vi "Revive Jaguars.vi"() -> ()   [LabVIEW 2011]
uses:
  <vilib>/Rock Robotics/WPI/CAN/Jaguar/SubVIs/WPI_CANJaguar_ControlMode.ctl
  <vilib>/Rock Robotics/WPI/CAN/Jaguar/SubVIs/WPI_CANJaguar_StatusSelect.ctl
  <vilib>/Rock Robotics/WPI/CAN/Jaguar/SubVIs/WPI_CANJaguar_SpeedReference.ctl
  Globals/Robot Jaguars.vi
  <vilib>/Rock Robotics/WPI/MotorControl/WPI_MotorControlOpenCANJaguar.vi
panel:
  out "FLD Mode":T1
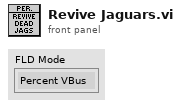
[diagram p1: front panel]
types:
  T1 = typedef "WPI_CANJaguar_ControlMode.ctl" = enum8{"Percent VBus", "Current", "Speed", "Position", "Voltage"}
  T2 = typedef "WPI_MotorControlDeviceRef.ctl" = cluster{"DeviceStatus":errorcluster, "Type":enum16{"PWM", "CAN"}, "PWM":cluster{"Digital Module":T3, "PWM Channel":T4, "DeadBand":T5}, "CAN":cluster{"Device Number":u8, "Control Mode":T1, "Semaphore":T6, "Max Vout":dbl}, "Invert":bool, "TransformRef":T7, "InvTransformRef":T7}
  T3 = typedef "FPGA_TypedefDigitalModule.ctl" = enum16{"Digital Module 1", "Digital Module 2"}
  T4 = typedef "FPGA_DIOPWMChannel.ctl" = enum8{"PWM 1", "PWM 2", "PWM 3", "PWM 4", "PWM 5", "PWM 6", "PWM 7", "PWM 8", "PWM 9", "PWM 10", "Invalid"}
  T5 = typedef "WPI_PWMDeadband.ctl" = cluster{"Name":string, "maxPositivePwm":i32, "minPositivePwm":i32, "centerPwm":i32, "maxNegativePwm":i32, "minNegativePwm":i32, "angularRange":u16}
  T6 = typedef "Semaphore RefNum" = refnum<k1>
  T7 = typedef "WPI_PWMTransform_ConPane.ctl" = refnum<vi>
  T8 = cluster{"Front Left Drive":T2, "Front Right Drive":T2, "Rear Left Drive":T2, "Rear Right Drive":T2, "Front Left Steer":T2, "Front Right Steer":T2, "Rear Left Steer":T2, "Rear Right Steer":T2}
  T9 = typedef "WPI_CANJaguar_StatusSelect.ctl" = enum16{"Output Percent VBus", "Output Voltage", "Bus Voltage", "Current", "Temperature", "Position", "Speed", "Limit Switches", "Faults", "Fault Counters", "Power Cycle"}
  T10 = typedef "WPI_CANJaguar_Status.ctl" = cluster{"Output Percent VBus":dbl, "Output Voltage":dbl, "Bus Voltage":dbl, "Current":dbl, "Temperature":dbl, "Position":dbl, "Speed":dbl, "Limits":cluster{"Forward Limit":bool, "Reverse Limit":bool, "Forward Soft Limit":bool, "Reverse Soft Limit":bool, "Sticky Forward Limit":bool, "Sticky Reverse Limit":bool, "Sticky Forward Soft Limit":bool, "Sticky Reverse Soft Limit":bool}, "Faults":cluster{"Current Fault":bool, "Temperature Fault":bool, "Bus Voltage Fault":bool, "Gate Driver Fault":bool, "Comm Fault":bool}, "Fault Counters":cluster{"Current Faults":u8, "Temperature Faults":u8, "Bus Voltage Faults":u8, "Gate Driver Faults":u8, "Comm Faults":u8, "CAN Status":u8, "CAN RX Errors":u8, "CAN TX Errors":u8}, "Power Cycle":bool}
  T11 = typedef "WPI_CANJaguar_SpeedReference.ctl" = u8
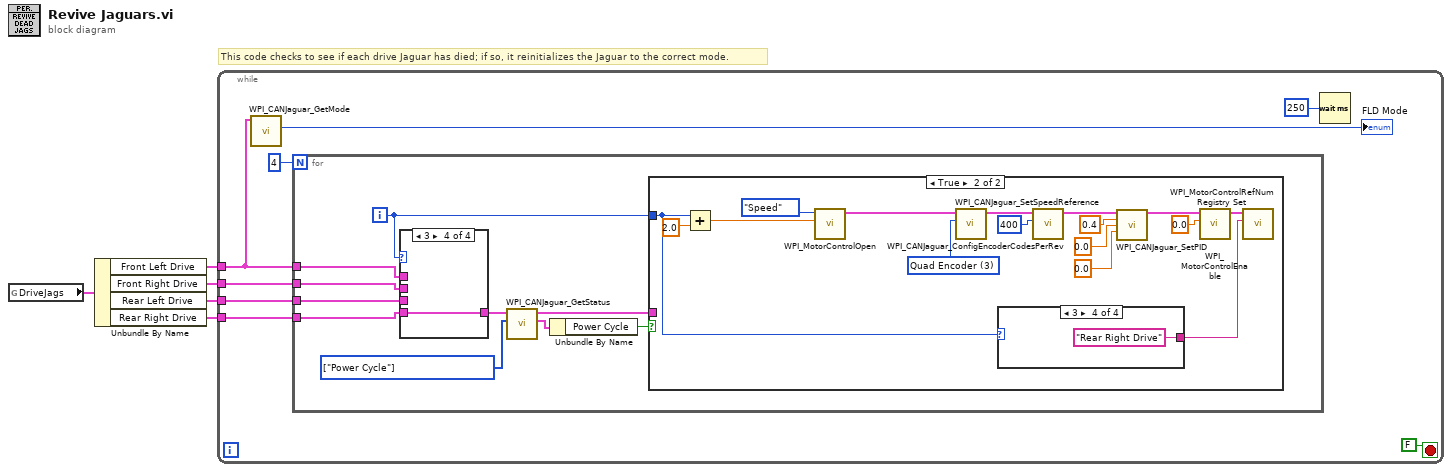
[diagram p0: block diagram]
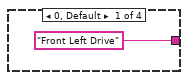
[diagram p3: hidden frame]
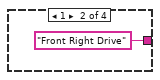
[diagram p4: hidden frame]
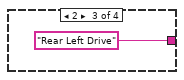
[diagram p5: hidden frame]
diagram:
  # "This code checks to see if each drive Jaguar has died; if so, it reinitializes the Jaguar to the correct mode."
  n1 = global read "Robot Jaguars.vi" "DriveJags"() -> (w1:T8)
  n2 = Unbundle By Name(w1) -> ("Front Left Drive"=w2:T2, "Front Right Drive"=w3:T2, "Rear Left Drive"=w4:T2, "Rear Right Drive"=w5:T2)
  n3 = while {
    tunnel: w2 -> [w7]
    tunnel: w3 -> [w10]
    tunnel: w4 -> [w9]
    tunnel: w5 -> [w8]
    stop <- FALSE stop-if-true
    n4 = call <vilib>:"WPI_CANJaguar_GetMode.vi"("CAN Jaguar Ref"=w7) -> ("Control Mode"=→"FLD Mode":T1)  [unwired: 8 in, 2 out]
    n5 = for {
      N: 4 -> [_]
      tunnel: w7 -> [w23]
      tunnel: w10 -> [w22]
      tunnel: w9 -> [w21]
      tunnel: w8 -> [w20]
      i -> [w14]
      w18 = T9[] [enum."Power Cycle"] items=["Output Percent VBus", "Output Voltage", "Bus Voltage", "Current", "Temperature", "Position", "Speed", "Limit Switches", "Faults", "Fault Counters", "Power Cycle"] ("Status Select")
      n6 = case shown="3" w14 {
        tunnel: w23 -> [w44 _ _ _]
        tunnel: w22 -> [_ w45 _ _]
        tunnel: w21 -> [_ _ w46 _]
        tunnel: w20 -> [_ _ _ w47]
        tunnel: [w44 w45 w46 w47] -> w19
        frame 0, Default {
        }
        frame 1 {
        }
        frame 2 {
        }
        frame 3 {
        }
      }
      n7 = call <vilib>:"WPI_CANJaguar_GetStatus.vi"("Status Select"=w18, "CAN Jaguar Ref"=w19) -> ("Status"=w17:T10, "CAN Jaguar Ref Out"=w15:T2)  [unwired: 7 in, 1 out]
      n8 = Unbundle By Name(w17) -> ("Power Cycle"=w16:bool)
      n9 = case shown="True" w16 {
        tunnel: w15 -> [_ _]
        tunnel: w14 -> [_ w27]
        frame False {
        }
        frame True {
          w34 = T11 3 items=["Encoder"=0, "Inv Encoder"=2, "Quad Encoder"=3, "None"=255] ("Speed Reference")
          n10 = Add(x=w27, y=2.0) -> (x+y=w29:dbl)
          n11 = call-poly <vilib>:"WPI_MotorControlOpen.vi"("Device Number"=w29, "Control Mode"=WPI_CANJaguar_ControlMode."Speed") -> ("MotorControlDeviceRef"=w24:T2)  [unwired: 8 in, 1 out]
          n12 = call <vilib>:"WPI_CANJaguar_SetSpeedReference.vi"("Speed Reference"=w34, "CAN Jaguar Ref"=w24) -> ("CAN Jaguar Ref Out"=w38:T2)  [unwired: 8 in, 1 out]
          n13 = case shown="3" w27 {
            tunnel: ["Front Left Drive" ("Jag Refnum Name") "Front Right Drive" ("Jag Refnum Name") "Rear Left Drive" ("Jag Refnum Name") "Rear Right Drive" ("Jag Refnum Name")] -> w26
            frame 0, Default {
            }
            frame 1 {
            }
            frame 2 {
            }
            frame 3 {
            }
          }
          n14 = call <vilib>:"WPI_CANJaguar_ConfigEncoderCodesPerRev.vi"("Encoder Codes Per Rev"=u16 400, "CAN Jaguar Ref"=w38) -> ("CAN Jaguar Ref Out"=w36:T2)  [unwired: 8 in, 1 out]
          n15 = call <vilib>:"WPI_CANJaguar_SetPID.vi"("CAN Jaguar Ref"=w36, "P"=0.4, "I"=0.0, "D"=0.0) -> ("CAN Jaguar Ref Out"=w35:T2)  [unwired: 10 in, 1 out]
          n16 = call <vilib>:"WPI_MotorControlEnable.vi"("Encoder Initial Position"=0.0, "CAN Jaguar Ref"=w35) -> ("CAN Jaguar Ref Out"=w25:T2)  [unwired: 8 in, 1 out]
          n17 = call <vilib>:"WPI_MotorControlRefNum Registry Set.vi"("refnum name"=w26, "MotorControlDevRef"=w25) -> ()  [unwired: 8 in, 2 out]
        }
      }
    }
    n18 = Wait (ms)(milliseconds to wait=u32 250) -> ()  [unwired: 1 out]
  }
